vi "BRig_RT__Case_Exp__State_initTrial__LC_Select__v10.vi"(6 "input_arrTrig":bool[](array[boolean]), 8 "input_dataTrial":u16[][](array[numeric]), 9 "input_dataExp":u16[](array[numeric]), 10 "input_dataLC":u16[](array[numeric]), 11 "input_dataCurrent":u16[](array[numeric])) -> (0 "output_dataTrial":u16[][](array[numeric]), 3 "output_dataCurrent":u16[](array[numeric]), 4 "output_arrTrig":bool[](array[boolean]))   [LabVIEW 2014]
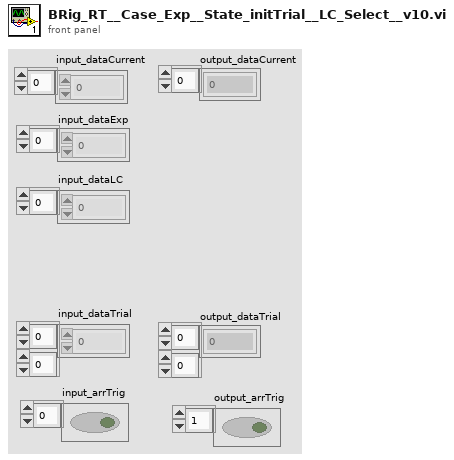
[diagram p1: front panel]
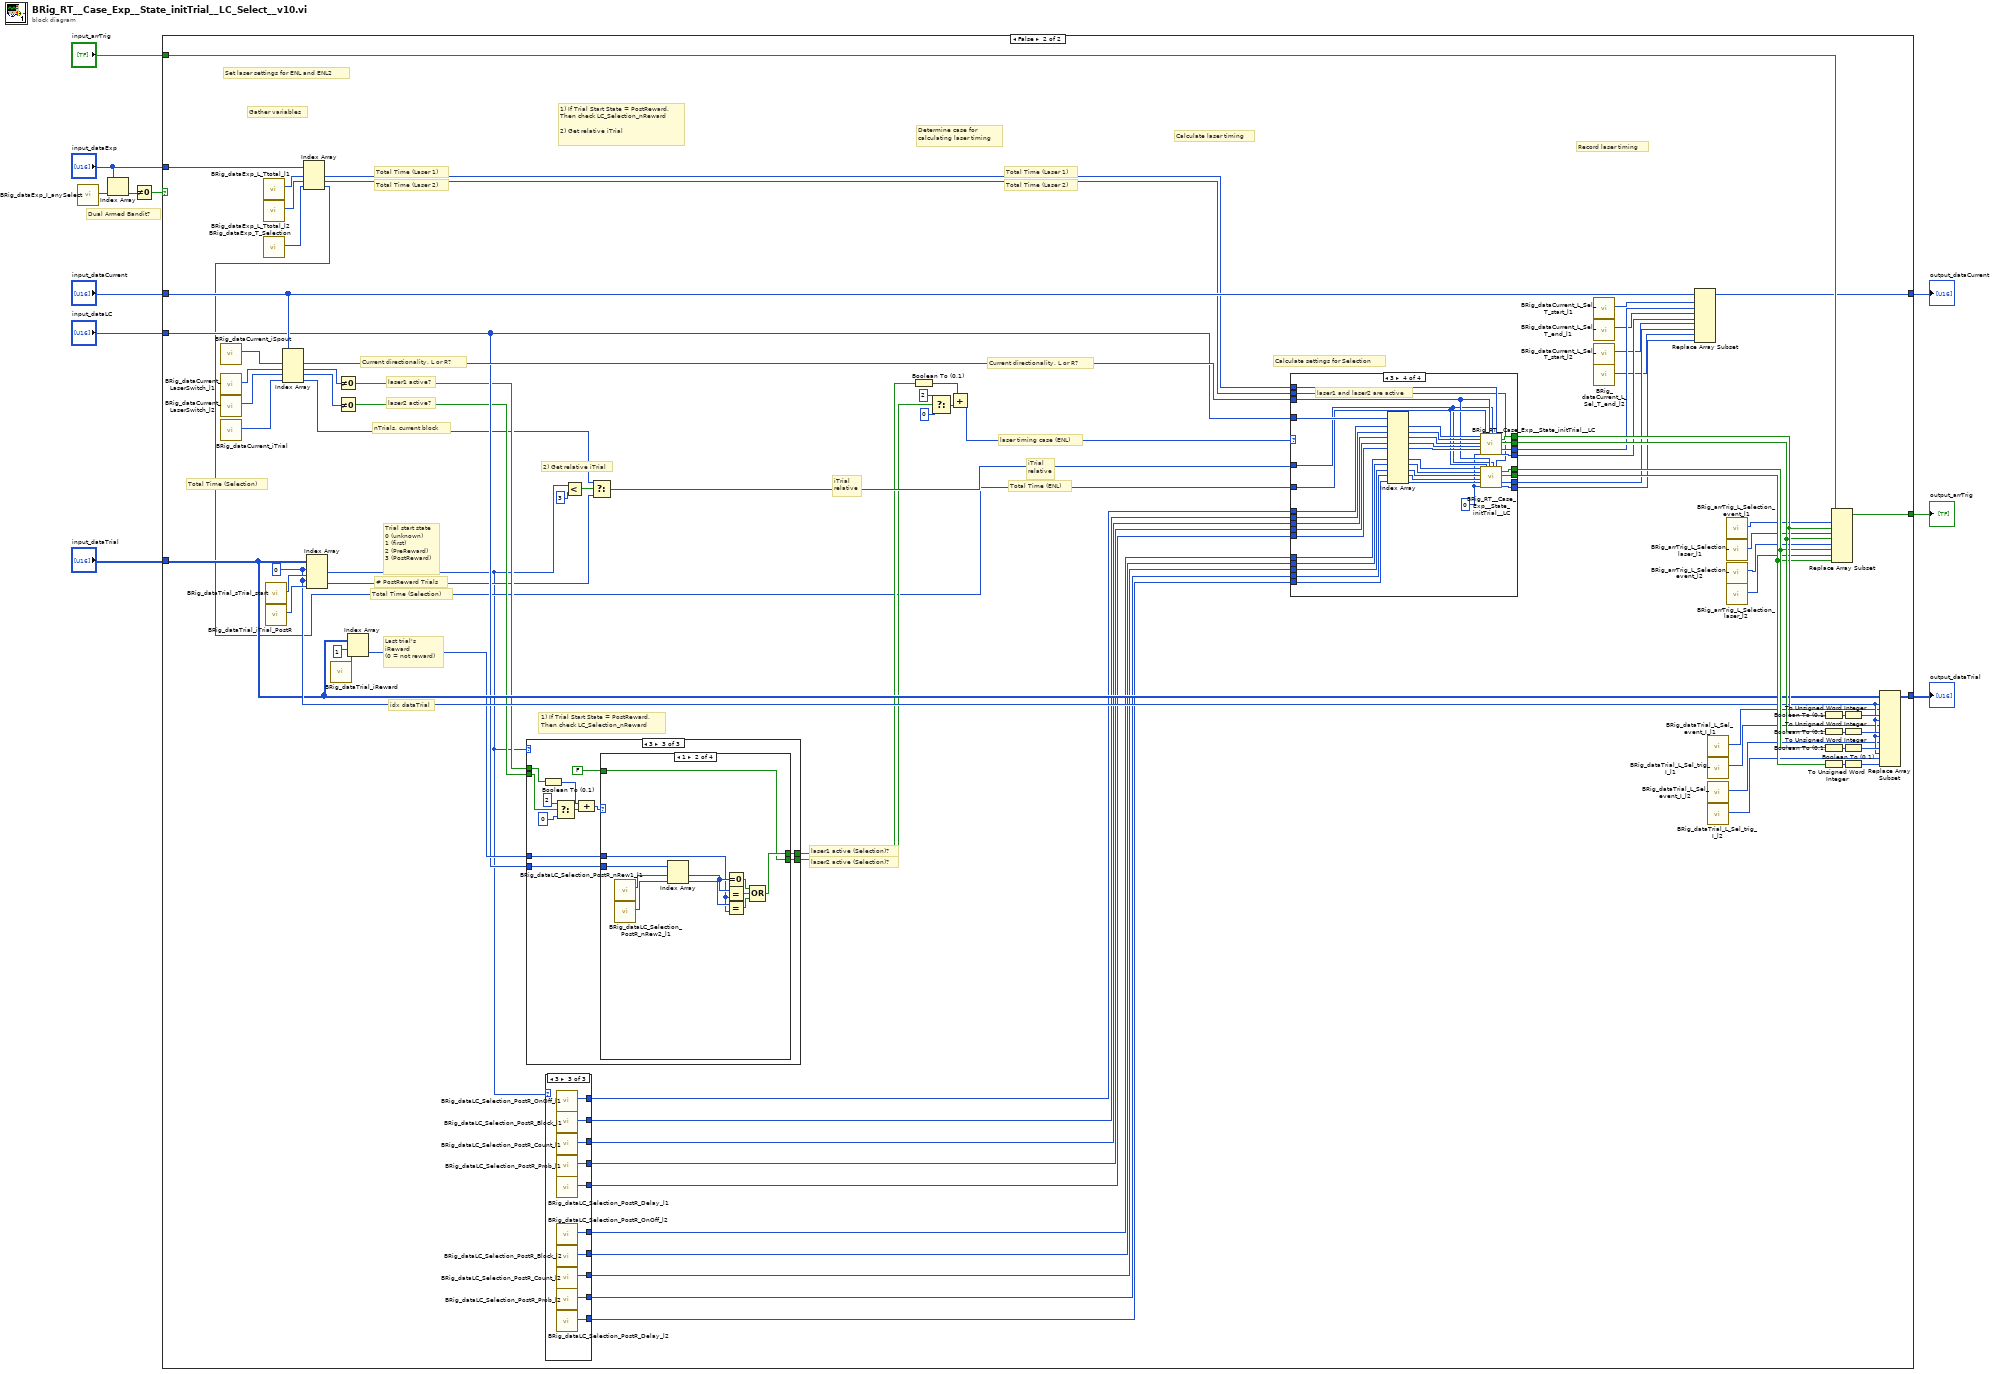
[diagram p0: block diagram]
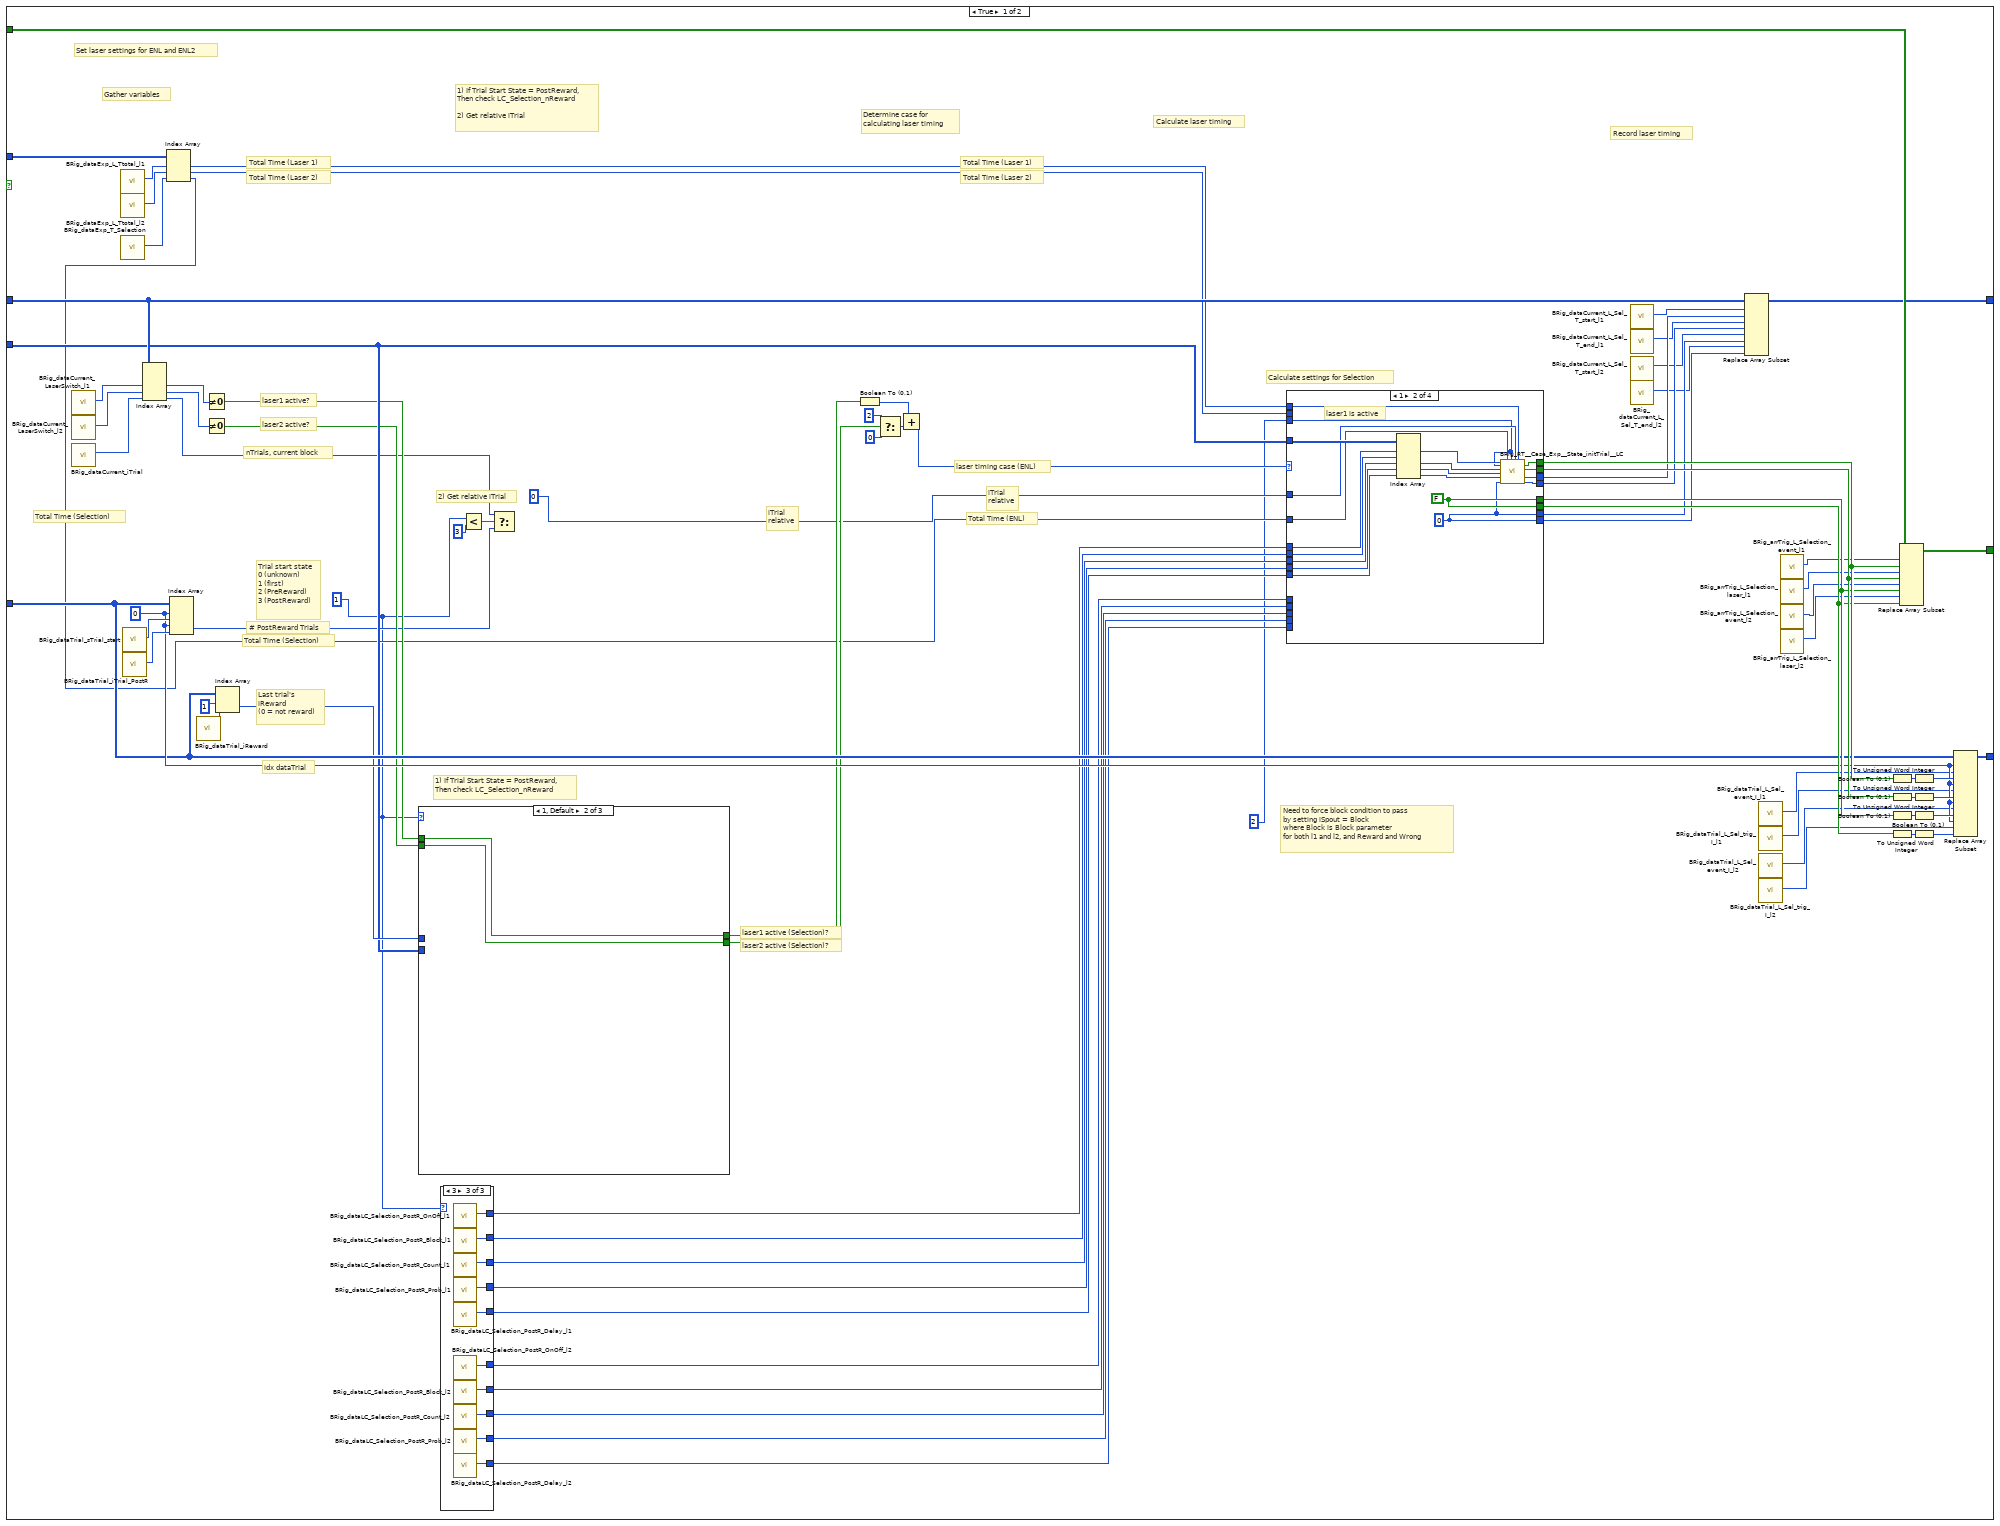
[diagram p2: hidden frame]
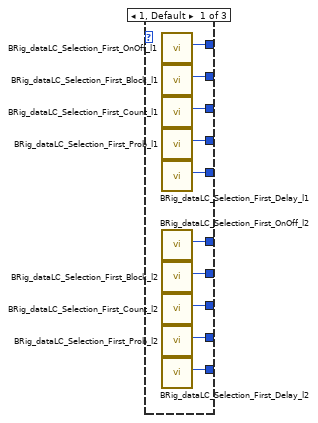
[diagram p3: hidden frame]
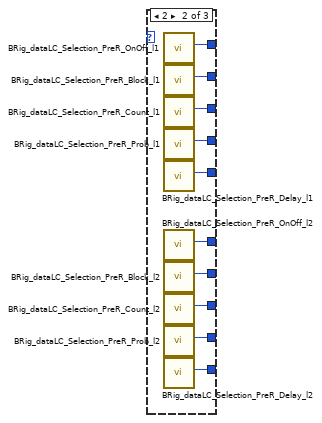
[diagram p4: hidden frame]
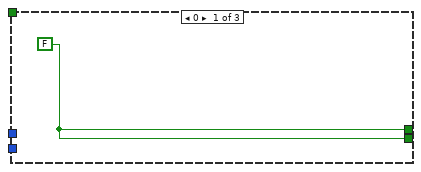
[diagram p5: hidden frame]
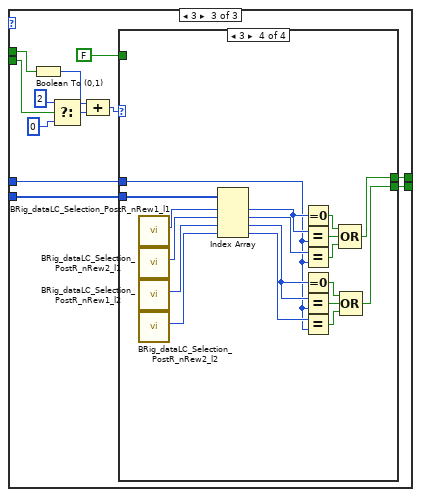
[diagram p6: hidden frame]
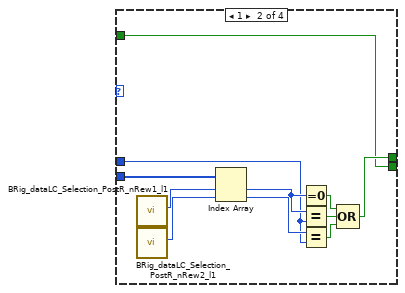
[diagram p8: hidden frame]
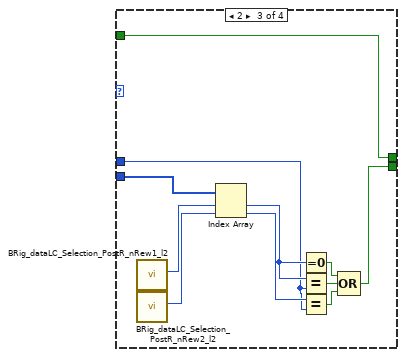
[diagram p9: hidden frame]
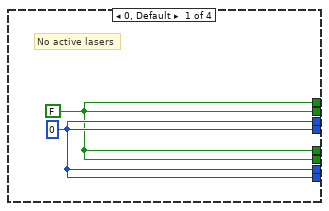
[diagram p10: hidden frame]
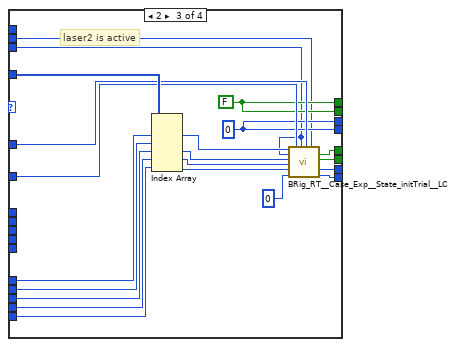
[diagram p11: hidden frame]
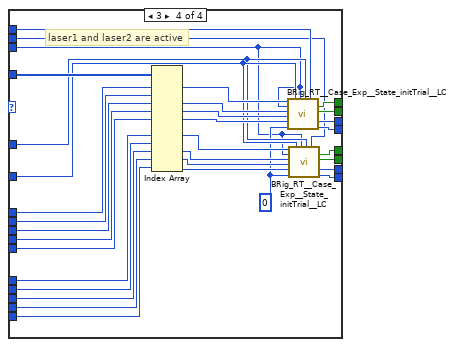
[diagram p12: hidden frame]
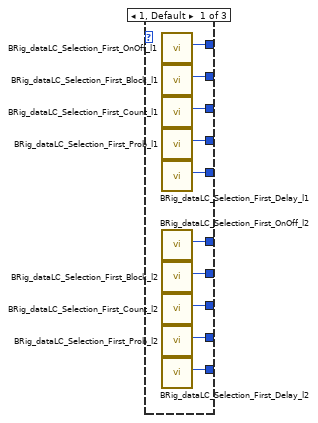
[diagram p13: hidden frame]
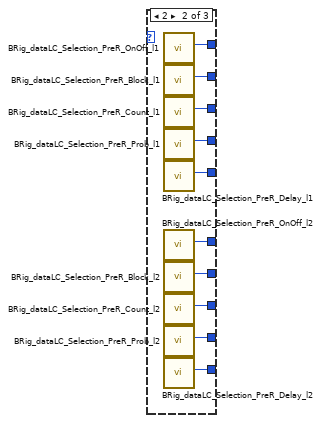
[diagram p14: hidden frame]
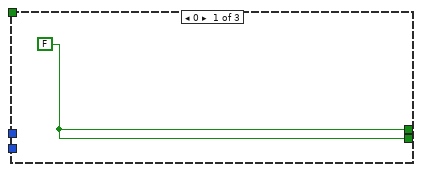
[diagram p15: hidden frame]
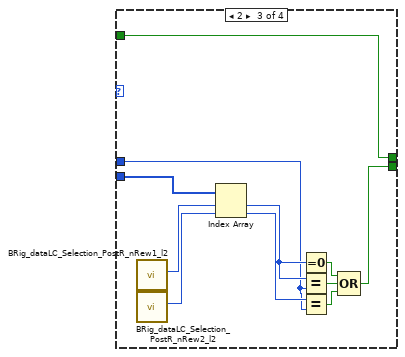
[diagram p18: hidden frame]
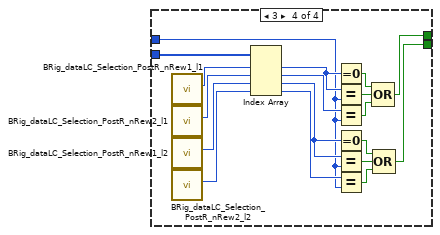
[diagram p19: hidden frame]
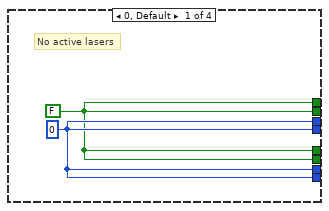
[diagram p20: hidden frame]
diagram:
  # "Dual Armed Bandit?"
  n1 = call "BRig_dataExp_I_anySelect.vi"() -> ("output_I_anySelect"=w4:i32)  [unwired: 11 in]
  n2 = Index Array(array="input_dataExp", index=w4) -> (element=w3:u16)
  n3 = Not Equal To 0?(x=w3) -> (x != 0?=w1:bool)
  n4 = case shown="False" w1 {
    tunnel: "input_arrTrig" -> [w81 w322]
    tunnel: [w80 w321] -> w10
    tunnel: [w67 w308] -> w9
    tunnel: "input_dataCurrent" -> [w66 w307]
    tunnel: [w65 w306] -> w7
    tunnel: "input_dataExp" -> [w58 w299]
    tunnel: "input_dataTrial" -> [w50 w290]
    tunnel: "input_dataLC" -> [w48 w288]
    frame True {
      w13 = u16 1
      w55 = 0
      # "Need to force block condition to pass\nby setting iSpout = Block\nwhere Block is Block parameter\nfor both l1 and l2, and Reward and Wrong"
      # "Total Time (Selection)"
      # "Record laser timing"
      # "Calculate laser timing"
      # "Total Time (ENL)"
      # "iTrial\nrelative"
      # "Total Time (Laser 2)"
      # "Total Time (Laser 1)"
      # "Determine case for\ncalculating laser timing"
      # "2) Get relative iTrial"
      # "1) If Trial Start State = PostReward,\nThen check LC_Selection_nReward"
      # "laser2 active (Selection)?"
      # "laser1 active (Selection)?"
      # "1) If Trial Start State = PostReward,\nThen check LC_Selection_nReward\n\n2) Get relative iTrial"
      # "Gather variables"
      # "Last trial's\niReward\n(0 = not reward)"
      # "nTrials, current block"
      # "idx dataTrial"
      # "Total Time (Selection)"
      # "# PostReward Trials"
      # "Total Time (Laser 2)"
      # "Total Time (Laser 1)"
      # "Calculate settings for Selection"
      # "Set laser settings for ENL and ENL2"
      # "iTrial\nrelative"
      # "laser timing case (ENL)"
      # "Trial start state\n0 (unknown)\n1 (first)\n2 (PreReward)\n3 (PostReward)"
      # "laser2 active?"
      # "laser1 active?"
      n5 = call "BRig_dataCurrent_LaserSwitch_l1.vi"() -> ("output_LaserSwitch_l1"=w90:i32)  [unwired: 11 in]
      n6 = call "BRig_dataCurrent_LaserSwitch_l2.vi"() -> ("output_LaserSwitch_l2"=w89:i32)  [unwired: 11 in]
      n7 = call "BRig_dataCurrent_iTrial.vi"() -> ("output_iTrial"=w56:i32)  [unwired: 11 in]
      n8 = call "BRig_dataExp_L_Ttotal_l1.vi"() -> ("output_L_Ttotal_l1"=w59:i32)  [unwired: 11 in]
      n9 = call "BRig_dataExp_L_Ttotal_l2.vi"() -> ("output_L_Ttotal_l2"=w60:i32)  [unwired: 11 in]
      n10 = call "BRig_dataExp_T_Selection.vi"() -> ("output_T_Selection"=w38:i32)  [unwired: 11 in]
      n11 = call "BRig_dataTrial_sTrial_start.vi"() -> ("output_sTrial_start"=w86:i32)  [unwired: 11 in]
      n12 = call "BRig_dataTrial_iTrial_PostR.vi"() -> ("output_iTrial_PostR"=w57:i32)  [unwired: 11 in]
      n13 = Index Array(array=w66, index #2=w90, index #3=w89, index #4=w56) -> (element #2=w88:u16, element #3=w87:u16, element #4=w43:u16)  [unwired: 1 in, 1 out]
      n14 = Index Array(array=w58, index #1=w59, index #2=w60, index #3=w38) -> (element #1=w54:u16, element #2=w53:u16, element #3=w37:u16)
      n15 = Index Array(array=w50, index (row) #1=w55, index (col) #1=w86, index (row) #2=w55, index (col) #2=w57) -> (element #2=w42:u16)  [unwired: 1 out]
      n16 = call "BRig_dataTrial_iReward.vi"() -> ("output_iReward"=w51:i32)  [unwired: 11 in]
      n17 = Not Equal To 0?(x=w88) -> (x != 0?=w46:bool)
      n18 = Not Equal To 0?(x=w87) -> (x != 0?=w47:bool)
      n19 = Index Array(array=w50, index (row)=1 ("disabled index (row)"), index (col)=w51) -> (element=w49:u16)
      n20 = case shown="1, Default" w13 {
        tunnel: w49 -> [_ _ w129]
        tunnel: w48 -> [_ _ w130]
        tunnel: w47 -> [_ w122 w124]
        tunnel: w46 -> [_ w123 w125]
        tunnel: [w121 w123 w128] -> w41
        tunnel: [w121 w122 w127] -> w40
        frame 0 {
          w121 = FALSE
        }
        frame 1, Default {
        }
        frame 3 {
          n21 = Boolean To (0,1)(Boolean=w125) -> (0, 1=w132:i16)
          n22 = Select(t=i16 2, s=w124, f=i16 0) -> (s? t:f=w133:i16)
          n23 = Compound Arithmetic op=ADD(w132, w133) -> (w131:i16)
          n24 = case shown="3" w131 {
            tunnel: w130 -> [_ w142 w153 w166]
            tunnel: w129 -> [_ w141 w152 w165]
            tunnel: [w136 w140 w150 w164] -> w128
            tunnel: [w136 w139 w151 w163] -> w127
            tunnel: FALSE -> [w136 w139 w150 _]
            frame 0, Default {
            }
            frame 1 {
              n25 = call "BRig_dataLC_Selection_PostR_nRew1_l1.vi"() -> ("output_Selection_PostR_nRew1_l1"=w137:i32)  [unwired: 11 in]
              n26 = call "BRig_dataLC_Selection_PostR_nRew2_l1.vi"() -> ("output_Selection_PostR_nRew2_l1"=w138:i32)  [unwired: 11 in]
              n27 = Index Array(array=w142, index #1=w137, index #2=w138) -> (element #1=w144:u16, element #2=w143:u16)
              n28 = Equal To 0?(x=w144) -> (x = 0?=w145:bool)
              n29 = Equal?(x=w144, y=w141) -> (x = y?=w146:bool)
              n30 = Equal?(x=w143, y=w141) -> (x = y?=w147:bool)
              n31 = Compound Arithmetic op=OR(w145, w146, w147) -> (w140:bool)
            }
            frame 2 {
              n32 = call "BRig_dataLC_Selection_PostR_nRew1_l2.vi"() -> ("output_Selection_PostR_nRew1_l2"=w148:i32)  [unwired: 11 in]
              n33 = call "BRig_dataLC_Selection_PostR_nRew2_l2.vi"() -> ("output_Selection_PostR_nRew2_l2"=w149:i32)  [unwired: 11 in]
              n34 = Index Array(array=w153, index #1=w148, index #2=w149) -> (element #1=w154:u16, element #2=w155:u16)
              n35 = Equal To 0?(x=w154) -> (x = 0?=w157:bool)
              n36 = Equal?(x=w154, y=w152) -> (x = y?=w156:bool)
              n37 = Equal?(x=w155, y=w152) -> (x = y?=w158:bool)
              n38 = Compound Arithmetic op=OR(w157, w156, w158) -> (w151:bool)
            }
            frame 3 {
              n39 = call "BRig_dataLC_Selection_PostR_nRew1_l1.vi"() -> ("output_Selection_PostR_nRew1_l1"=w159:i32)  [unwired: 11 in]
              n40 = call "BRig_dataLC_Selection_PostR_nRew2_l1.vi"() -> ("output_Selection_PostR_nRew2_l1"=w160:i32)  [unwired: 11 in]
              n41 = call "BRig_dataLC_Selection_PostR_nRew1_l2.vi"() -> ("output_Selection_PostR_nRew1_l2"=w161:i32)  [unwired: 11 in]
              n42 = call "BRig_dataLC_Selection_PostR_nRew2_l2.vi"() -> ("output_Selection_PostR_nRew2_l2"=w162:i32)  [unwired: 11 in]
              n43 = Index Array(array=w166, index #1=w159, index #2=w160, index #3=w161, index #4=w162) -> (element #1=w170:u16, element #2=w169:u16, element #3=w167:u16, element #4=w168:u16)
              n44 = Equal To 0?(x=w170) -> (x = 0?=w171:bool)
              n45 = Equal?(x=w170, y=w165) -> (x = y?=w172:bool)
              n46 = Equal?(x=w169, y=w165) -> (x = y?=w173:bool)
              n47 = Equal To 0?(x=w167) -> (x = 0?=w175:bool)
              n48 = Equal?(x=w167, y=w165) -> (x = y?=w174:bool)
              n49 = Equal?(x=w168, y=w165) -> (x = y?=w176:bool)
              n50 = Compound Arithmetic op=OR(w171, w172, w173) -> (w164:bool)
              n51 = Compound Arithmetic op=OR(w175, w174, w176) -> (w163:bool)
            }
          }
        }
      }
      n52 = case shown="3" w13 {
        tunnel: [w100 w110 w120] -> w36
        tunnel: [w93 w108 w118] -> w35
        tunnel: [w94 w107 w117] -> w34
        tunnel: [w95 w106 w116] -> w33
        tunnel: [w96 w105 w115] -> w32
        tunnel: [w99 w109 w119] -> w31
        tunnel: [w97 w104 w114] -> w30
        tunnel: [w98 w103 w113] -> w29
        tunnel: [w91 w102 w112] -> w28
        tunnel: [w92 w101 w111] -> w27
        frame 1, Default {
          n53 = call "BRig_dataLC_Selection_First_OnOff_l1.vi"() -> ("output_Selection_First_OnOff"=w100:i32)  [unwired: 11 in]
          n54 = call "BRig_dataLC_Selection_First_Block_l1.vi"() -> ("output_Selection_First_Block"=w93:i32)  [unwired: 11 in]
          n55 = call "BRig_dataLC_Selection_First_Count_l1.vi"() -> ("output_Selection_First_Count"=w94:i32)  [unwired: 11 in]
          n56 = call "BRig_dataLC_Selection_First_Prob_l1.vi"() -> ("output_Selection_First_Prob"=w95:i32)  [unwired: 11 in]
          n57 = call "BRig_dataLC_Selection_First_Delay_l1.vi"() -> ("output_Selection_First_Delay"=w96:i32)  [unwired: 11 in]
          n58 = call "BRig_dataLC_Selection_First_OnOff_l2.vi"() -> ("output_Selection_First_OnOff_l2"=w99:i32)  [unwired: 11 in]
          n59 = call "BRig_dataLC_Selection_First_Block_l2.vi"() -> ("output_Selection_First_Block_l2"=w97:i32)  [unwired: 11 in]
          n60 = call "BRig_dataLC_Selection_First_Count_l2.vi"() -> ("output_Selection_First_Count_l2"=w98:i32)  [unwired: 11 in]
          n61 = call "BRig_dataLC_Selection_First_Prob_l2.vi"() -> ("output_Selection_First_Prob_l2"=w91:i32)  [unwired: 11 in]
          n62 = call "BRig_dataLC_Selection_First_Delay_l2.vi"() -> ("output_Selection_First_Delay_l2"=w92:i32)  [unwired: 11 in]
        }
        frame 2 {
          n63 = call "BRig_dataLC_Selection_PreR_OnOff_l1.vi"() -> ("output_Selection_PreR_OnOff"=w110:i32)  [unwired: 11 in]
          n64 = call "BRig_dataLC_Selection_PreR_Block_l1.vi"() -> ("output_Selection_PreR_Block"=w108:i32)  [unwired: 11 in]
          n65 = call "BRig_dataLC_Selection_PreR_Count_l1.vi"() -> ("output_Selection_PreR_Count"=w107:i32)  [unwired: 11 in]
          n66 = call "BRig_dataLC_Selection_PreR_Prob_l1.vi"() -> ("output_Selection_PreR_Prob"=w106:i32)  [unwired: 11 in]
          n67 = call "BRig_dataLC_Selection_PreR_Delay_l1.vi"() -> ("output_Selection_PreR_Delay"=w105:i32)  [unwired: 11 in]
          n68 = call "BRig_dataLC_Selection_PreR_OnOff_l2.vi"() -> ("output_Selection_PreR_OnOff_l2"=w109:i32)  [unwired: 11 in]
          n69 = call "BRig_dataLC_Selection_PreR_Block_l2.vi"() -> ("output_Selection_PreR_Block_l2"=w104:i32)  [unwired: 11 in]
          n70 = call "BRig_dataLC_Selection_PreR_Count_l2.vi"() -> ("output_Selection_PreR_Count_l2"=w103:i32)  [unwired: 11 in]
          n71 = call "BRig_dataLC_Selection_PreR_Prob_l2.vi"() -> ("output_Selection_PreR_Prob_l2"=w102:i32)  [unwired: 11 in]
          n72 = call "BRig_dataLC_Selection_PreR_Delay_l2.vi"() -> ("output_Selection_PreR_Delay_l2"=w101:i32)  [unwired: 11 in]
        }
        frame 3 {
          n73 = call "BRig_dataLC_Selection_PostR_OnOff_l1.vi"() -> ("output_Selection_PostR_OnOff"=w120:i32)  [unwired: 11 in]
          n74 = call "BRig_dataLC_Selection_PostR_Block_l1.vi"() -> ("output_Selection_PostR_Block"=w118:i32)  [unwired: 11 in]
          n75 = call "BRig_dataLC_Selection_PostR_Count_l1.vi"() -> ("output_Selection_PostR_Count"=w117:i32)  [unwired: 11 in]
          n76 = call "BRig_dataLC_Selection_PostR_Prob_l1.vi"() -> ("output_Selection_PostR_Prob"=w116:i32)  [unwired: 11 in]
          n77 = call "BRig_dataLC_Selection_PostR_Delay_l1.vi"() -> ("output_Selection_PostR_Delay"=w115:i32)  [unwired: 11 in]
          n78 = call "BRig_dataLC_Selection_PostR_OnOff_l2.vi"() -> ("output_Selection_PostR_OnOff_l2"=w119:i32)  [unwired: 11 in]
          n79 = call "BRig_dataLC_Selection_PostR_Block_l2.vi"() -> ("output_Selection_PostR_Block_l2"=w114:i32)  [unwired: 11 in]
          n80 = call "BRig_dataLC_Selection_PostR_Count_l2.vi"() -> ("output_Selection_PostR_Count_l2"=w113:i32)  [unwired: 11 in]
          n81 = call "BRig_dataLC_Selection_PostR_Prob_l2.vi"() -> ("output_Selection_PostR_Prob_l2"=w112:i32)  [unwired: 11 in]
          n82 = call "BRig_dataLC_Selection_PostR_Delay_l2.vi"() -> ("output_Selection_PostR_Delay_l2"=w111:i32)  [unwired: 11 in]
        }
      }
      n83 = Less?(x=w13, y=u16 3) -> (x < y?=w44:bool)
      n84 = Select(t=w43, s=w44, f=w42) -> ()  [unwired: 1 out]
      n85 = Boolean To (0,1)(Boolean=w41) -> (0, 1=w83:i16)
      n86 = Select(t=i16 2, s=w40, f=i16 0) -> (s? t:f=w84:i16)
      n87 = Add(x=w83, y=w84) -> (x+y=w39:i16)
      n88 = case shown="1" w39 {
        tunnel: w48 -> [_ w198 w219 w252]
        tunnel: u16 2 ("input_sState_start") -> [_ w179 w199 w220]
        tunnel: w37 -> [_ w193 w214 w243]
        tunnel: u16 0 -> [_ w192 w213 w242]
        tunnel: [w177 w191 w203 w241] -> w75
        tunnel: [w177 w190 w203 w240] -> w72
        tunnel: [w178 w189 w202 w239] -> w64
        tunnel: [w178 w188 w202 w238] -> w63
        tunnel: [w177 w182 w212 w237] -> w68
        tunnel: [w178 w180 w211 w236] -> w62
        tunnel: [w177 w182 w210 w235] -> w70
        tunnel: [w178 w180 w209 w234] -> w61
        tunnel: w36 -> [_ w187 _ w233]
        tunnel: w35 -> [_ w186 _ w232]
        tunnel: w34 -> [_ w185 _ w231]
        tunnel: w33 -> [_ w184 _ w230]
        tunnel: w32 -> [_ w183 _ w229]
        tunnel: w31 -> [_ _ w208 w228]
        tunnel: w30 -> [_ _ w207 w227]
        tunnel: w29 -> [_ _ w206 w226]
        tunnel: w28 -> [_ _ w205 w225]
        tunnel: w27 -> [_ _ w204 w224]
        tunnel: w54 -> [_ w181 _ w223]
        tunnel: w53 -> [_ _ w201 w222]
        frame 0, Default {
          w178 = u16 0
          w177 = FALSE
          # "No active lasers"
        }
        frame 1 {
          w180 = u16 0
          w182 = FALSE
          # "laser1 is active"
          n89 = Index Array(array=w198, index #1=w187, index #2=w186, index #3=w185, index #4=w184, index #5=w183) -> (element #1=w197:u16, element #3=w196:u16, element #4=w195:u16, element #5=w194:u16)  [unwired: 1 out]
          n90 = call "BRig_RT__Case_Exp__State_initTrial__LC.vi"("input_L_OnOff"=w197, "input_L_Block"=w179, "input_L_Count"=w196, "input_L_Prob"=w195, "input_L_Tdelay"=w194, "input_L_delayOpt"=w180, "input_T_state"=w193, "input_iSpout"=w179, "input_iTrial_relative"=w192, "input_L_T"=w181) -> ("output_LC_Event"=w191:bool, "output_LC_Laser"=w190:bool, "output_L_Tstart"=w189:u16, "output_L_Tend"=w188:u16)  [unwired: 6 in]
        }
        frame 2 {
          w202 = u16 0
          w203 = FALSE
          # "laser2 is active"
          n91 = Index Array(array=w219, index #1=w208, index #2=w207, index #3=w206, index #4=w205, index #5=w204) -> (element #1=w215:u16, element #3=w216:u16, element #4=w217:u16, element #5=w218:u16)  [unwired: 1 out]
          n92 = call "BRig_RT__Case_Exp__State_initTrial__LC.vi"("input_L_OnOff"=w215, "input_L_Block"=w199, "input_L_Count"=w216, "input_L_Prob"=w217, "input_L_Tdelay"=w218, "input_L_delayOpt"=u16 0, "input_T_state"=w214, "input_iSpout"=w199, "input_iTrial_relative"=w213, "input_L_T"=w201) -> ("output_LC_Event"=w210:bool, "output_LC_Laser"=w212:bool, "output_L_Tstart"=w211:u16, "output_L_Tend"=w209:u16)  [unwired: 6 in]
        }
        frame 3 {
          w221 = u16 0 ("input_L_delayOpt")
          # "laser1 and laser2 are active"
          n93 = Index Array(array=w252, index #1=w233, index #2=w232, index #3=w231, index #4=w230, index #5=w229, index #7=w228, index #8=w227, index #9=w226, index #10=w225, index #11=w224) -> (element #1=w251:u16, element #3=w250:u16, element #4=w249:u16, element #5=w248:u16, element #7=w244:u16, element #9=w245:u16, element #10=w246:u16, element #11=w247:u16)  [unwired: 1 in, 3 out]
          n94 = call "BRig_RT__Case_Exp__State_initTrial__LC.vi"("input_L_OnOff"=w251, "input_L_Block"=w220, "input_L_Count"=w250, "input_L_Prob"=w249, "input_L_Tdelay"=w248, "input_L_delayOpt"=w221, "input_T_state"=w243, "input_iSpout"=w220, "input_iTrial_relative"=w242, "input_L_T"=w223) -> ("output_LC_Event"=w241:bool, "output_LC_Laser"=w240:bool, "output_L_Tstart"=w239:u16, "output_L_Tend"=w238:u16)  [unwired: 6 in]
          n95 = call "BRig_RT__Case_Exp__State_initTrial__LC.vi"("input_L_OnOff"=w244, "input_L_Block"=w220, "input_L_Count"=w245, "input_L_Prob"=w246, "input_L_Tdelay"=w247, "input_L_delayOpt"=w221, "input_T_state"=w243, "input_iSpout"=w220, "input_iTrial_relative"=w242, "input_L_T"=w222) -> ("output_LC_Event"=w235:bool, "output_LC_Laser"=w237:bool, "output_L_Tstart"=w236:u16, "output_L_Tend"=w234:u16)  [unwired: 6 in]
        }
      }
      n96 = call "BRig_dataCurrent_L_Sel_T_start_l1.vi"() -> ("output_L_Sel_T_start_l1"=w23:i32)  [unwired: 11 in]
      n97 = call "BRig_dataCurrent_L_Sel_T_end_l1.vi"() -> ("output_L_Sel_T_end_l1"=w24:i32)  [unwired: 11 in]
      n98 = call "BRig_dataCurrent_L_Sel_T_start_l2.vi"() -> ("output_L_Sel_T_start_l2"=w25:i32)  [unwired: 11 in]
      n99 = call "BRig_dataCurrent_L_Sel_T_end_l2.vi"() -> ("output_L_Sel_T_end_l2"=w26:i32)  [unwired: 11 in]
      n100 = Replace Array Subset(array=w66, new element #1=w64, index #1=w23, new element #2=w63, index #2=w24, new element #3=w62, index #3=w25, new element #4=w61, index #4=w26) -> (w65:u16[])
      n101 = call "BRig_dataTrial_L_Sel_event_I_l1.vi"() -> ("output_L_Sel_event_I_l1"=w18:i32)  [unwired: 11 in]
      n102 = call "BRig_dataTrial_L_Sel_trig_I_l1.vi"() -> ("output_L_Sel_trig_I_l1"=w17:i32)  [unwired: 11 in]
      n103 = call "BRig_dataTrial_L_Sel_event_I_l2.vi"() -> ("output_L_Sel_event_I_l2"=w16:i32)  [unwired: 11 in]
      n104 = call "BRig_dataTrial_L_Sel_trig_I_l2.vi"() -> ("output_L_Sel_trig_I_l2"=w15:i32)  [unwired: 11 in]
      n105 = call "BRig_arrTrig_L_Selection_event_l1.vi"() -> ("output_L_Sel_event_l1"=w19:i32)  [unwired: 11 in]
      n106 = call "BRig_arrTrig_L_Selection_laser_l1.vi"() -> ("output_L_Sel_laserTrig_l1"=w20:i32)  [unwired: 11 in]
      n107 = call "BRig_arrTrig_L_Selection_event_l2.vi"() -> ("output_L_Sel_event_l2"=w21:i32)  [unwired: 11 in]
      n108 = call "BRig_arrTrig_L_Selection_laser_l2.vi"() -> ("output_L_Sel_laserTrig_l2"=w22:i32)  [unwired: 11 in]
      n109 = Boolean To (0,1)(Boolean=w75) -> (0, 1=w79:i16)
      n110 = Boolean To (0,1)(Boolean=w72) -> (0, 1=w78:i16)
      n111 = Boolean To (0,1)(Boolean=w70) -> (0, 1=w76:i16)
      n112 = Boolean To (0,1)(Boolean=w68) -> (0, 1=w77:i16)
      n113 = Replace Array Subset(array=w81, new element #1=w75, index #1=w19, new element #2=w72, index #2=w20, new element #3=w70, index #3=w21, new element #4=w68, index #4=w22) -> (w80:bool[])
      n114 = To Unsigned Word Integer(number=w79) -> (unsigned 16bit integer=w74:u16)
      n115 = To Unsigned Word Integer(number=w78) -> (unsigned 16bit integer=w73:u16)
      n116 = To Unsigned Word Integer(number=w76) -> (unsigned 16bit integer=w71:u16)
      n117 = To Unsigned Word Integer(number=w77) -> (unsigned 16bit integer=w69:u16)
      n118 = Replace Array Subset(array=w50, new element #1=w74, index (row) #1=w55, index (col) #1=w18, new element #2=w73, index (row) #2=w55, index (col) #2=w17, new element #3=w71, index (row) #3=w55, index (col) #3=w16, new element #4=w69, index (row) #4=w55, index (col) #4=w15) -> (w67:u16[][])
    }
    frame False {
      w296 = 0
      # "Total Time (Selection)"
      # "Record laser timing"
      # "Calculate laser timing"
      # "Total Time (ENL)"
      # "iTrial\nrelative"
      # "Total Time (Laser 2)"
      # "Total Time (Laser 1)"
      # "Current directionality, L or R?"
      # "Determine case for\ncalculating laser timing"
      # "2) Get relative iTrial"
      # "1) If Trial Start State = PostReward,\nThen check LC_Selection_nReward"
      # "laser2 active (Selection)?"
      # "laser1 active (Selection)?"
      # "1) If Trial Start State = PostReward,\nThen check LC_Selection_nReward\n\n2) Get relative iTrial"
      # "Gather variables"
      # "Last trial's\niReward\n(0 = not reward)"
      # "nTrials, current block"
      # "idx dataTrial"
      # "Total Time (Selection)"
      # "# PostReward Trials"
      # "Current directionality, L or R?"
      # "Total Time (Laser 2)"
      # "Total Time (Laser 1)"
      # "Calculate settings for Selection"
      # "Set laser settings for ENL and ENL2"
      # "iTrial\nrelative"
      # "laser timing case (ENL)"
      # "Trial start state\n0 (unknown)\n1 (first)\n2 (PreReward)\n3 (PostReward)"
      # "laser2 active?"
      # "laser1 active?"
      n119 = call "BRig_dataCurrent_iSpout.vi"() -> ("output_iSpout"=w323:i32)  [unwired: 11 in]
      n120 = call "BRig_dataCurrent_LaserSwitch_l1.vi"() -> ("output_LaserSwitch_l1"=w332:i32)  [unwired: 11 in]
      n121 = call "BRig_dataCurrent_LaserSwitch_l2.vi"() -> ("output_LaserSwitch_l2"=w331:i32)  [unwired: 11 in]
      n122 = call "BRig_dataCurrent_iTrial.vi"() -> ("output_iTrial"=w297:i32)  [unwired: 11 in]
      n123 = call "BRig_dataExp_L_Ttotal_l1.vi"() -> ("output_L_Ttotal_l1"=w300:i32)  [unwired: 11 in]
      n124 = call "BRig_dataExp_L_Ttotal_l2.vi"() -> ("output_L_Ttotal_l2"=w301:i32)  [unwired: 11 in]
      n125 = call "BRig_dataExp_T_Selection.vi"() -> ("output_T_Selection"=w277:i32)  [unwired: 11 in]
      n126 = call "BRig_dataTrial_sTrial_start.vi"() -> ("output_sTrial_start"=w328:i32)  [unwired: 11 in]
      n127 = call "BRig_dataTrial_iTrial_PostR.vi"() -> ("output_iTrial_PostR"=w298:i32)  [unwired: 11 in]
      n128 = Index Array(array=w307, index #1=w323, index #2=w332, index #3=w331, index #4=w297) -> (element #1=w293:u16, element #2=w330:u16, element #3=w329:u16, element #4=w283:u16)
      n129 = Index Array(array=w299, index #1=w300, index #2=w301, index #3=w277) -> (element #1=w295:u16, element #2=w294:u16, element #3=w276:u16)
      n130 = Index Array(array=w290, index (row) #1=w296, index (col) #1=w328, index (row) #2=w296, index (col) #2=w298) -> (element #1=w275:u16, element #2=w282:u16)
      n131 = call "BRig_dataTrial_iReward.vi"() -> ("output_iReward"=w291:i32)  [unwired: 11 in]
      n132 = Not Equal To 0?(x=w330) -> (x != 0?=w286:bool)
      n133 = Not Equal To 0?(x=w329) -> (x != 0?=w287:bool)
      n134 = Index Array(array=w290, index (row)=1 ("disabled index (row)"), index (col)=w291) -> (element=w289:u16)
      n135 = case shown="3" w275 {
        tunnel: w289 -> [_ _ w371]
        tunnel: w288 -> [_ _ w372]
        tunnel: w287 -> [_ w364 w366]
        tunnel: w286 -> [_ w365 w367]
        tunnel: [w363 w365 w370] -> w280
        tunnel: [w363 w364 w369] -> w279
        frame 0 {
          w363 = FALSE
        }
        frame 1, Default {
        }
        frame 3 {
          n136 = Boolean To (0,1)(Boolean=w367) -> (0, 1=w374:i16)
          n137 = Select(t=i16 2, s=w366, f=i16 0) -> (s? t:f=w375:i16)
          n138 = Compound Arithmetic op=ADD(w374, w375) -> (w373:i16)
          n139 = case shown="1" w373 {
            tunnel: w372 -> [_ w384 w395 w408]
            tunnel: w371 -> [_ w383 w394 w407]
            tunnel: [w378 w382 w392 w406] -> w370
            tunnel: [w378 w381 w393 w405] -> w369
            tunnel: FALSE -> [w378 w381 w392 _]
            frame 0, Default {
            }
            frame 1 {
              n140 = call "BRig_dataLC_Selection_PostR_nRew1_l1.vi"() -> ("output_Selection_PostR_nRew1_l1"=w379:i32)  [unwired: 11 in]
              n141 = call "BRig_dataLC_Selection_PostR_nRew2_l1.vi"() -> ("output_Selection_PostR_nRew2_l1"=w380:i32)  [unwired: 11 in]
              n142 = Index Array(array=w384, index #1=w379, index #2=w380) -> (element #1=w386:u16, element #2=w385:u16)
              n143 = Equal To 0?(x=w386) -> (x = 0?=w387:bool)
              n144 = Equal?(x=w386, y=w383) -> (x = y?=w388:bool)
              n145 = Equal?(x=w385, y=w383) -> (x = y?=w389:bool)
              n146 = Compound Arithmetic op=OR(w387, w388, w389) -> (w382:bool)
            }
            frame 2 {
              n147 = call "BRig_dataLC_Selection_PostR_nRew1_l2.vi"() -> ("output_Selection_PostR_nRew1_l2"=w390:i32)  [unwired: 11 in]
              n148 = call "BRig_dataLC_Selection_PostR_nRew2_l2.vi"() -> ("output_Selection_PostR_nRew2_l2"=w391:i32)  [unwired: 11 in]
              n149 = Index Array(array=w395, index #1=w390, index #2=w391) -> (element #1=w396:u16, element #2=w397:u16)
              n150 = Equal To 0?(x=w396) -> (x = 0?=w399:bool)
              n151 = Equal?(x=w396, y=w394) -> (x = y?=w398:bool)
              n152 = Equal?(x=w397, y=w394) -> (x = y?=w400:bool)
              n153 = Compound Arithmetic op=OR(w399, w398, w400) -> (w393:bool)
            }
            frame 3 {
              n154 = call "BRig_dataLC_Selection_PostR_nRew1_l1.vi"() -> ("output_Selection_PostR_nRew1_l1"=w401:i32)  [unwired: 11 in]
              n155 = call "BRig_dataLC_Selection_PostR_nRew2_l1.vi"() -> ("output_Selection_PostR_nRew2_l1"=w402:i32)  [unwired: 11 in]
              n156 = call "BRig_dataLC_Selection_PostR_nRew1_l2.vi"() -> ("output_Selection_PostR_nRew1_l2"=w403:i32)  [unwired: 11 in]
              n157 = call "BRig_dataLC_Selection_PostR_nRew2_l2.vi"() -> ("output_Selection_PostR_nRew2_l2"=w404:i32)  [unwired: 11 in]
              n158 = Index Array(array=w408, index #1=w401, index #2=w402, index #3=w403, index #4=w404) -> (element #1=w412:u16, element #2=w411:u16, element #3=w409:u16, element #4=w410:u16)
              n159 = Equal To 0?(x=w412) -> (x = 0?=w413:bool)
              n160 = Equal?(x=w412, y=w407) -> (x = y?=w414:bool)
              n161 = Equal?(x=w411, y=w407) -> (x = y?=w415:bool)
              n162 = Equal To 0?(x=w409) -> (x = 0?=w417:bool)
              n163 = Equal?(x=w409, y=w407) -> (x = y?=w416:bool)
              n164 = Equal?(x=w410, y=w407) -> (x = y?=w418:bool)
              n165 = Compound Arithmetic op=OR(w413, w414, w415) -> (w406:bool)
              n166 = Compound Arithmetic op=OR(w417, w416, w418) -> (w405:bool)
            }
          }
        }
      }
      n167 = case shown="3" w275 {
        tunnel: [w342 w352 w362] -> w274
        tunnel: [w335 w350 w353] -> w273
        tunnel: [w336 w349 w360] -> w272
        tunnel: [w337 w348 w359] -> w271
        tunnel: [w338 w347 w358] -> w270
        tunnel: [w341 w351 w361] -> w269
        tunnel: [w339 w346 w357] -> w268
        tunnel: [w340 w345 w356] -> w267
        tunnel: [w333 w344 w355] -> w266
        tunnel: [w334 w343 w354] -> w265
        frame 1, Default {
          n168 = call "BRig_dataLC_Selection_First_OnOff_l1.vi"() -> ("output_Selection_First_OnOff"=w342:i32)  [unwired: 11 in]
          n169 = call "BRig_dataLC_Selection_First_Block_l1.vi"() -> ("output_Selection_First_Block"=w335:i32)  [unwired: 11 in]
          n170 = call "BRig_dataLC_Selection_First_Count_l1.vi"() -> ("output_Selection_First_Count"=w336:i32)  [unwired: 11 in]
          n171 = call "BRig_dataLC_Selection_First_Prob_l1.vi"() -> ("output_Selection_First_Prob"=w337:i32)  [unwired: 11 in]
          n172 = call "BRig_dataLC_Selection_First_Delay_l1.vi"() -> ("output_Selection_First_Delay"=w338:i32)  [unwired: 11 in]
          n173 = call "BRig_dataLC_Selection_First_OnOff_l2.vi"() -> ("output_Selection_First_OnOff_l2"=w341:i32)  [unwired: 11 in]
          n174 = call "BRig_dataLC_Selection_First_Block_l2.vi"() -> ("output_Selection_First_Block_l2"=w339:i32)  [unwired: 11 in]
          n175 = call "BRig_dataLC_Selection_First_Count_l2.vi"() -> ("output_Selection_First_Count_l2"=w340:i32)  [unwired: 11 in]
          n176 = call "BRig_dataLC_Selection_First_Prob_l2.vi"() -> ("output_Selection_First_Prob_l2"=w333:i32)  [unwired: 11 in]
          n177 = call "BRig_dataLC_Selection_First_Delay_l2.vi"() -> ("output_Selection_First_Delay_l2"=w334:i32)  [unwired: 11 in]
        }
        frame 2 {
          n178 = call "BRig_dataLC_Selection_PreR_OnOff_l1.vi"() -> ("output_Selection_PreR_OnOff"=w352:i32)  [unwired: 11 in]
          n179 = call "BRig_dataLC_Selection_PreR_Block_l1.vi"() -> ("output_Selection_PreR_Block"=w350:i32)  [unwired: 11 in]
          n180 = call "BRig_dataLC_Selection_PreR_Count_l1.vi"() -> ("output_Selection_PreR_Count"=w349:i32)  [unwired: 11 in]
          n181 = call "BRig_dataLC_Selection_PreR_Prob_l1.vi"() -> ("output_Selection_PreR_Prob"=w348:i32)  [unwired: 11 in]
          n182 = call "BRig_dataLC_Selection_PreR_Delay_l1.vi"() -> ("output_Selection_PreR_Delay"=w347:i32)  [unwired: 11 in]
          n183 = call "BRig_dataLC_Selection_PreR_OnOff_l2.vi"() -> ("output_Selection_PreR_OnOff_l2"=w351:i32)  [unwired: 11 in]
          n184 = call "BRig_dataLC_Selection_PreR_Block_l2.vi"() -> ("output_Selection_PreR_Block_l2"=w346:i32)  [unwired: 11 in]
          n185 = call "BRig_dataLC_Selection_PreR_Count_l2.vi"() -> ("output_Selection_PreR_Count_l2"=w345:i32)  [unwired: 11 in]
          n186 = call "BRig_dataLC_Selection_PreR_Prob_l2.vi"() -> ("output_Selection_PreR_Prob_l2"=w344:i32)  [unwired: 11 in]
          n187 = call "BRig_dataLC_Selection_PreR_Delay_l2.vi"() -> ("output_Selection_PreR_Delay_l2"=w343:i32)  [unwired: 11 in]
        }
        frame 3 {
          n188 = call "BRig_dataLC_Selection_PostR_OnOff_l1.vi"() -> ("output_Selection_PostR_OnOff"=w362:i32)  [unwired: 11 in]
          n189 = call "BRig_dataLC_Selection_PostR_Block_l1.vi"() -> ("output_Selection_PostR_Block"=w353:i32)  [unwired: 11 in]
          n190 = call "BRig_dataLC_Selection_PostR_Count_l1.vi"() -> ("output_Selection_PostR_Count"=w360:i32)  [unwired: 11 in]
          n191 = call "BRig_dataLC_Selection_PostR_Prob_l1.vi"() -> ("output_Selection_PostR_Prob"=w359:i32)  [unwired: 11 in]
          n192 = call "BRig_dataLC_Selection_PostR_Delay_l1.vi"() -> ("output_Selection_PostR_Delay"=w358:i32)  [unwired: 11 in]
          n193 = call "BRig_dataLC_Selection_PostR_OnOff_l2.vi"() -> ("output_Selection_PostR_OnOff_l2"=w361:i32)  [unwired: 11 in]
          n194 = call "BRig_dataLC_Selection_PostR_Block_l2.vi"() -> ("output_Selection_PostR_Block_l2"=w357:i32)  [unwired: 11 in]
          n195 = call "BRig_dataLC_Selection_PostR_Count_l2.vi"() -> ("output_Selection_PostR_Count_l2"=w356:i32)  [unwired: 11 in]
          n196 = call "BRig_dataLC_Selection_PostR_Prob_l2.vi"() -> ("output_Selection_PostR_Prob_l2"=w355:i32)  [unwired: 11 in]
          n197 = call "BRig_dataLC_Selection_PostR_Delay_l2.vi"() -> ("output_Selection_PostR_Delay_l2"=w354:i32)  [unwired: 11 in]
        }
      }
      n198 = Less?(x=w275, y=u16 3) -> (x < y?=w284:bool)
      n199 = Select(t=w283, s=w284, f=w282) -> (s? t:f=w281:u16)
      n200 = Boolean To (0,1)(Boolean=w280) -> (0, 1=w325:i16)
      n201 = Select(t=i16 2, s=w279, f=i16 0) -> (s? t:f=w326:i16)
      n202 = Add(x=w325, y=w326) -> (x+y=w278:i16)
      n203 = case shown="3" w278 {
        tunnel: w288 -> [_ w441 w463 w498]
        tunnel: w293 -> [_ w434 w456 w486]
        tunnel: w276 -> [_ w435 w457 w487]
        tunnel: w281 -> [_ w433 w455 w485]
        tunnel: [w419 w432 w445 w484] -> w316
        tunnel: [w419 w431 w445 w483] -> w313
        tunnel: [w420 w430 w444 w482] -> w305
        tunnel: [w420 w429 w444 w481] -> w304
        tunnel: [w419 w423 w454 w480] -> w309
        tunnel: [w420 w421 w453 w479] -> w303
        tunnel: [w419 w423 w452 w478] -> w311
        tunnel: [w420 w421 w451 w477] -> w302
        tunnel: w274 -> [_ w428 _ w476]
        tunnel: w273 -> [_ w427 _ w475]
        tunnel: w272 -> [_ w426 _ w474]
        tunnel: w271 -> [_ w425 _ w473]
        tunnel: w270 -> [_ w424 _ w472]
        tunnel: w269 -> [_ _ w450 w471]
        tunnel: w268 -> [_ _ w449 w470]
        tunnel: w267 -> [_ _ w448 w469]
        tunnel: w266 -> [_ _ w447 w468]
        tunnel: w265 -> [_ _ w446 w467]
        tunnel: w295 -> [_ w422 _ w466]
        tunnel: w294 -> [_ _ w443 w465]
        frame 0, Default {
          w420 = u16 0
          w419 = FALSE
          # "No active lasers"
        }
        frame 1 {
          w421 = u16 0
          w423 = FALSE
          # "laser1 is active"
          n204 = Index Array(array=w441, index #1=w428, index #2=w427, index #3=w426, index #4=w425, index #5=w424) -> (element #1=w440:u16, element #2=w439:u16, element #3=w438:u16, element #4=w437:u16, element #5=w436:u16)
          n205 = call "BRig_RT__Case_Exp__State_initTrial__LC.vi"("input_L_OnOff"=w440, "input_L_Block"=w439, "input_L_Count"=w438, "input_L_Prob"=w437, "input_L_Tdelay"=w436, "input_L_delayOpt"=w421, "input_T_state"=w435, "input_iSpout"=w434, "input_iTrial_relative"=w433, "input_L_T"=w422) -> ("output_LC_Event"=w432:bool, "output_LC_Laser"=w431:bool, "output_L_Tstart"=w430:u16, "output_L_Tend"=w429:u16)  [unwired: 6 in]
        }
        frame 2 {
          w444 = u16 0
          w445 = FALSE
          # "laser2 is active"
          n206 = Index Array(array=w463, index #1=w450, index #2=w449, index #3=w448, index #4=w447, index #5=w446) -> (element #1=w458:u16, element #2=w459:u16, element #3=w460:u16, element #4=w461:u16, element #5=w462:u16)
          n207 = call "BRig_RT__Case_Exp__State_initTrial__LC.vi"("input_L_OnOff"=w458, "input_L_Block"=w459, "input_L_Count"=w460, "input_L_Prob"=w461, "input_L_Tdelay"=w462, "input_L_delayOpt"=u16 0, "input_T_state"=w457, "input_iSpout"=w456, "input_iTrial_relative"=w455, "input_L_T"=w443) -> ("output_LC_Event"=w452:bool, "output_LC_Laser"=w454:bool, "output_L_Tstart"=w453:u16, "output_L_Tend"=w451:u16)  [unwired: 6 in]
        }
        frame 3 {
          w464 = u16 0 ("input_L_delayOpt")
          # "laser1 and laser2 are active"
          n208 = Index Array(array=w498, index #1=w476, index #2=w475, index #3=w474, index #4=w473, index #5=w472, index #7=w471, index #8=w470, index #9=w469, index #10=w468, index #11=w467) -> (element #1=w497:u16, element #2=w496:u16, element #3=w495:u16, element #4=w494:u16, element #5=w493:u16, element #7=w488:u16, element #8=w489:u16, element #9=w490:u16, element #10=w491:u16, element #11=w492:u16)  [unwired: 1 in, 1 out]
          n209 = call "BRig_RT__Case_Exp__State_initTrial__LC.vi"("input_L_OnOff"=w497, "input_L_Block"=w496, "input_L_Count"=w495, "input_L_Prob"=w494, "input_L_Tdelay"=w493, "input_L_delayOpt"=w464, "input_T_state"=w487, "input_iSpout"=w486, "input_iTrial_relative"=w485, "input_L_T"=w466) -> ("output_LC_Event"=w484:bool, "output_LC_Laser"=w483:bool, "output_L_Tstart"=w482:u16, "output_L_Tend"=w481:u16)  [unwired: 6 in]
          n210 = call "BRig_RT__Case_Exp__State_initTrial__LC.vi"("input_L_OnOff"=w488, "input_L_Block"=w489, "input_L_Count"=w490, "input_L_Prob"=w491, "input_L_Tdelay"=w492, "input_L_delayOpt"=w464, "input_T_state"=w487, "input_iSpout"=w486, "input_iTrial_relative"=w485, "input_L_T"=w465) -> ("output_LC_Event"=w478:bool, "output_LC_Laser"=w480:bool, "output_L_Tstart"=w479:u16, "output_L_Tend"=w477:u16)  [unwired: 6 in]
        }
      }
      n211 = call "BRig_dataCurrent_L_Sel_T_start_l1.vi"() -> ("output_L_Sel_T_start_l1"=w261:i32)  [unwired: 11 in]
      n212 = call "BRig_dataCurrent_L_Sel_T_end_l1.vi"() -> ("output_L_Sel_T_end_l1"=w262:i32)  [unwired: 11 in]
      n213 = call "BRig_dataCurrent_L_Sel_T_start_l2.vi"() -> ("output_L_Sel_T_start_l2"=w263:i32)  [unwired: 11 in]
      n214 = call "BRig_dataCurrent_L_Sel_T_end_l2.vi"() -> ("output_L_Sel_T_end_l2"=w264:i32)  [unwired: 11 in]
      n215 = Replace Array Subset(array=w307, new element #1=w305, index #1=w261, new element #2=w304, index #2=w262, new element #3=w303, index #3=w263, new element #4=w302, index #4=w264) -> (w306:u16[])
      n216 = call "BRig_dataTrial_L_Sel_event_I_l1.vi"() -> ("output_L_Sel_event_I_l1"=w256:i32)  [unwired: 11 in]
      n217 = call "BRig_dataTrial_L_Sel_trig_I_l1.vi"() -> ("output_L_Sel_trig_I_l1"=w255:i32)  [unwired: 11 in]
      n218 = call "BRig_dataTrial_L_Sel_event_I_l2.vi"() -> ("output_L_Sel_event_I_l2"=w254:i32)  [unwired: 11 in]
      n219 = call "BRig_dataTrial_L_Sel_trig_I_l2.vi"() -> ("output_L_Sel_trig_I_l2"=w253:i32)  [unwired: 11 in]
      n220 = call "BRig_arrTrig_L_Selection_event_l1.vi"() -> ("output_L_Sel_event_l1"=w257:i32)  [unwired: 11 in]
      n221 = call "BRig_arrTrig_L_Selection_laser_l1.vi"() -> ("output_L_Sel_laserTrig_l1"=w258:i32)  [unwired: 11 in]
      n222 = call "BRig_arrTrig_L_Selection_event_l2.vi"() -> ("output_L_Sel_event_l2"=w259:i32)  [unwired: 11 in]
      n223 = call "BRig_arrTrig_L_Selection_laser_l2.vi"() -> ("output_L_Sel_laserTrig_l2"=w260:i32)  [unwired: 11 in]
      n224 = Boolean To (0,1)(Boolean=w316) -> (0, 1=w320:i16)
      n225 = Boolean To (0,1)(Boolean=w313) -> (0, 1=w319:i16)
      n226 = Boolean To (0,1)(Boolean=w311) -> (0, 1=w317:i16)
      n227 = Boolean To (0,1)(Boolean=w309) -> (0, 1=w318:i16)
      n228 = Replace Array Subset(array=w322, new element #1=w316, index #1=w257, new element #2=w313, index #2=w258, new element #3=w311, index #3=w259, new element #4=w309, index #4=w260) -> (w321:bool[])
      n229 = To Unsigned Word Integer(number=w320) -> (unsigned 16bit integer=w315:u16)
      n230 = To Unsigned Word Integer(number=w319) -> (unsigned 16bit integer=w314:u16)
      n231 = To Unsigned Word Integer(number=w317) -> (unsigned 16bit integer=w312:u16)
      n232 = To Unsigned Word Integer(number=w318) -> (unsigned 16bit integer=w310:u16)
      n233 = Replace Array Subset(array=w290, new element #1=w315, index (row) #1=w296, index (col) #1=w256, new element #2=w314, index (row) #2=w296, index (col) #2=w255, new element #3=w312, index (row) #3=w296, index (col) #3=w254, new element #4=w310, index (row) #4=w296, index (col) #4=w253) -> (w308:u16[][])
    }
  }
  "output_dataCurrent" <- w7
  "output_arrTrig" <- w10
  "output_dataTrial" <- w9
